vi "Read Channel Setting.vi"(8 "error in (no error)":errorcluster) -> (0 "error out":errorcluster, 3 "Channel Setting":T1(array[cluster]))   [LabVIEW 2017]
uses:
  <vilib>/Utility/file.llb/Read Delimited Spreadsheet (string).vi
panel:
  out "subarray":string[][](array[string])
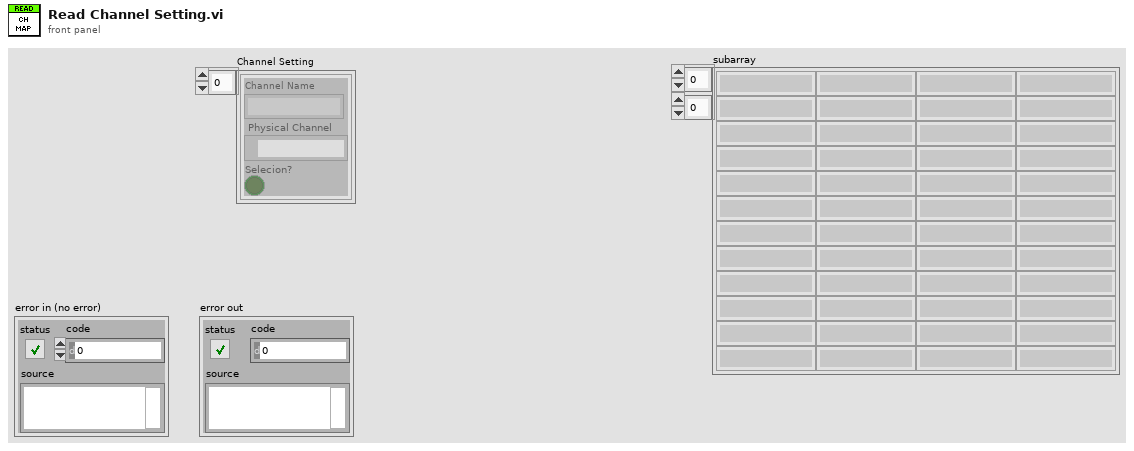
[diagram p1: front panel]
types:
  T1 = cluster{"Channel Name":string, " Physical Channel":tag, "Selecion?":bool}[]
  T2 = cluster{"Channel Name":string, " Physical Channel":tag, "Selecion?":bool}
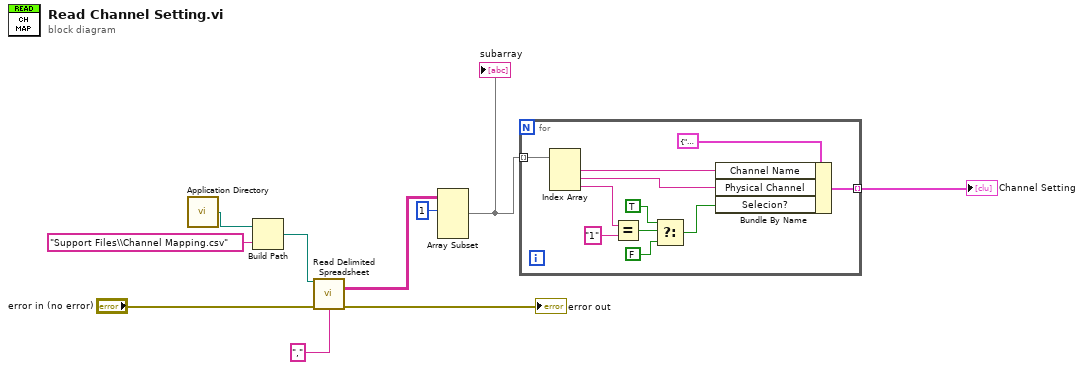
[diagram p0: block diagram]
diagram:
  n1 = call <vilib>:"Application Directory.vi"() -> ("Application Directory"=w9:path)
  n2 = Build Path(base path=w9, name or relative path="Support Files\\Channel Mapping.csv") -> (appended path=w7:path)
  n3 = call-poly <vilib>:"Read Delimited Spreadsheet.vi"("file path (dialog if empty)"=w7, "error in (no error)"="error in (no error)", "delimiter (\\t)"="," ("delimiter (\\t)")) -> ("all rows"=w2:string[][], "error out"=→"error out":errorcluster)  [unwired: 7 in, 4 out]
  n4 = Array Subset(array=w2, index (row)=1 ("index")) -> (w1:string[][])  [unwired: 3 in]
  "subarray" <- w1
  n5 = for {
    tunnel: w1 -> [w21] mode=indexing
    tunnel: [w11] -> w10 mode=indexing
    n6 = Index Array(array=w21) -> (element #1=w19:string, element #2=w18:string, element #3=w17:string)  [unwired: 3 in]
    n7 = Equal?(x=w17, y="1") -> (x = y?=w15:bool)
    n8 = Select(t=TRUE, s=w15, f=FALSE) -> (s? t:f=w12:bool)
    n9 = Bundle By Name(cluster=T2 {"Channel Name"="", " Physical Channel"="", "Selecion?"=FALSE} ("Channel Mapping"), "Channel Name"=w19, "Physical Channel"=w18, "Selecion?"=w12) -> (w11:T2)
  }
  "Channel Setting" <- w10
